vi "Execution End.vi"(8 "error in (no error)":errorcluster, 10 "Execution in":refnum<data-value>, 11 "JsonReportPlugin in":refnum<class "JsonReportPlugin.lvclass">) -> (0 "error out":errorcluster, 2 "Execution out":refnum<data-value>, 3 "JsonReportPlugin out":refnum<class "JsonReportPlugin.lvclass">)   [LabVIEW 2015, in "JsonReportPlugin.lvclass"]
uses:
  JsonReportPlugin.lvclass
  Core/Execution.lvclass
  Core/Step.lvclass
panel:
  out "resulting string":string
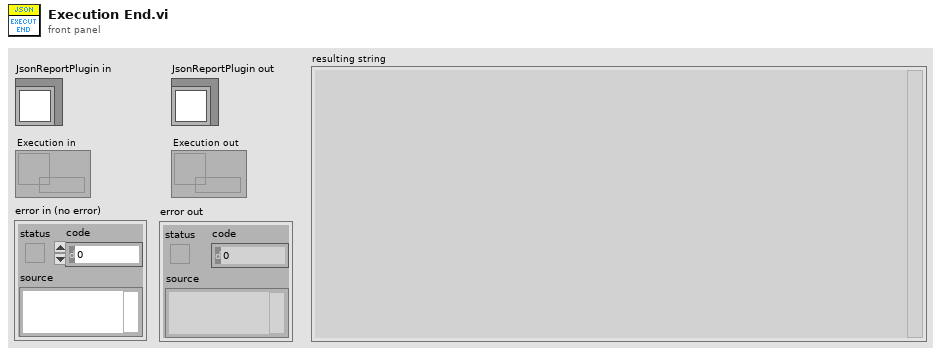
[diagram p1: front panel]
types:
  T1 = typedef "Execution.lvclass/EXECUTION_CONTEXT.ctl" = cluster{"Continue Test":bool, "DUT Info":T2, "StartTime":timestamp, "EndTime":timestamp, "Result":T3, "Info Text":string, "ResultList":T4[]}
  T2 = typedef "Execution.lvclass/DUT_INFO_TYPEDEF.ctl" = cluster{"SN":string, "Model":string, "PartNumber":string, "Revision":string, "Software":string, "Hardware":string}
  T3 = typedef "Execution.lvclass/EXECUTION_RESULT_TYPEDEF.ctl" = enum16{"Unknow", "Terminated", "Passed", "Failed", "Error"}
  T4 = typedef "Execution.lvclass/STEP_RESULT.ctl" = cluster{"StepIndex":u32, "Step":refnum<class "Step.lvclass">, "StartTime":timestamp, "EndTime":timestamp, "Result":T5, "Error Info":string, "Measure Results":T6[]}
  T5 = typedef "Step.lvclass/STEP_STATUS.ctl" = enum16{"Skipped", "Done", "Passed", "Failed", "Error"}
  T6 = typedef "Execution.lvclass/STEP_MEASURE_RESULT.ctl" = cluster{"Name":string, "Data Type":T7, "Check Type":T8, "String Limit":string, "Lower Limit":dbl, "Upper Limit":dbl, "Boolean Limit":bool, "Ignore Case":bool, "Measure Data":variant, "Result":T5, "Error Info":string}
  T7 = typedef "Step.lvclass/OUTPUT_DATA_TYPE.ctl" = enum16{"Boolean", "String", "Numeric", "Other"}
  T8 = typedef "Step.lvclass/OUTPUT_CHECK_TYPE.ctl" = enum16{"INVALID", "DO_NOT_CHECK", "RECORD", "VARIABLE", "EQUAL", "NOT_EQUAL", "STR_CONTAINS", "STR_START_WITH", "STR_END_WITH", "STR_REGEX_MATCH", "NUM_GT", "NUM_LT", "NUM_GE", "NUM_LE", "NUM_RANGE", "NUM_RANGE_BDY"}
  T9 = typedef "STATION_INFO_TYPEDEF.ctl" = cluster{"Process":string, "Station Name":string, "Fixture":string, "Production Line":string, "Factory":string}
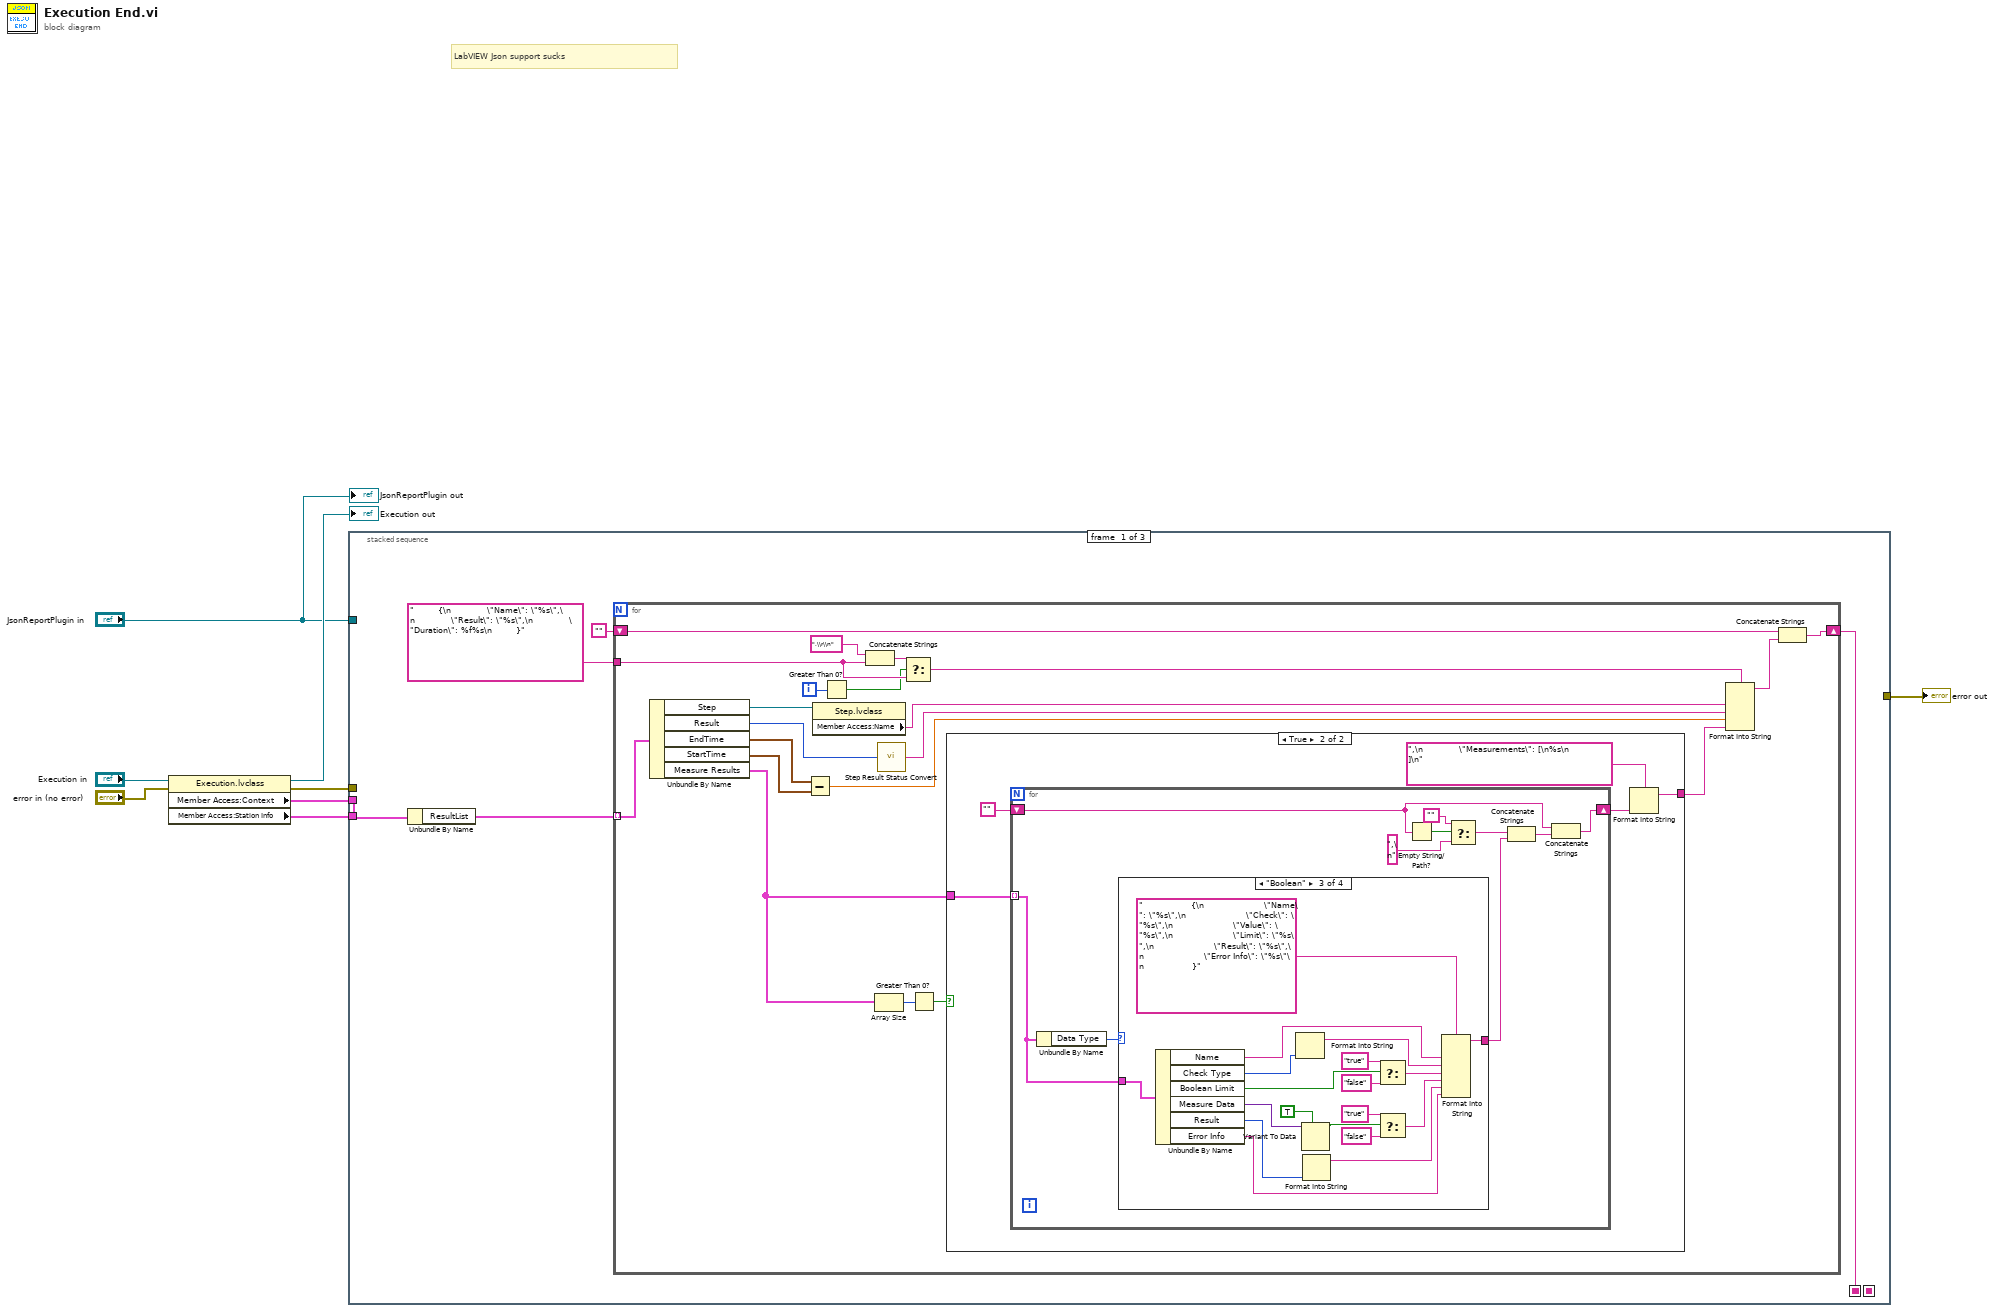
[diagram p0: block diagram]
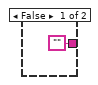
[diagram p2: hidden frame]
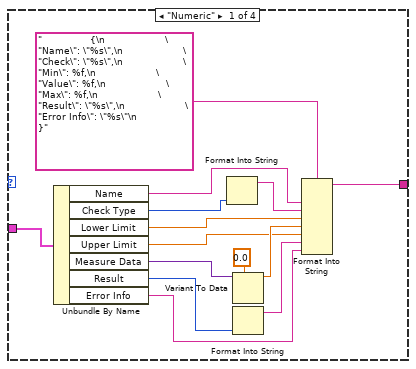
[diagram p3: hidden frame]
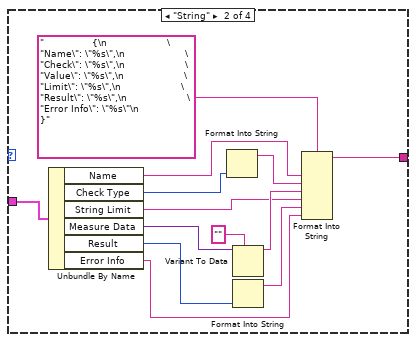
[diagram p4: hidden frame]
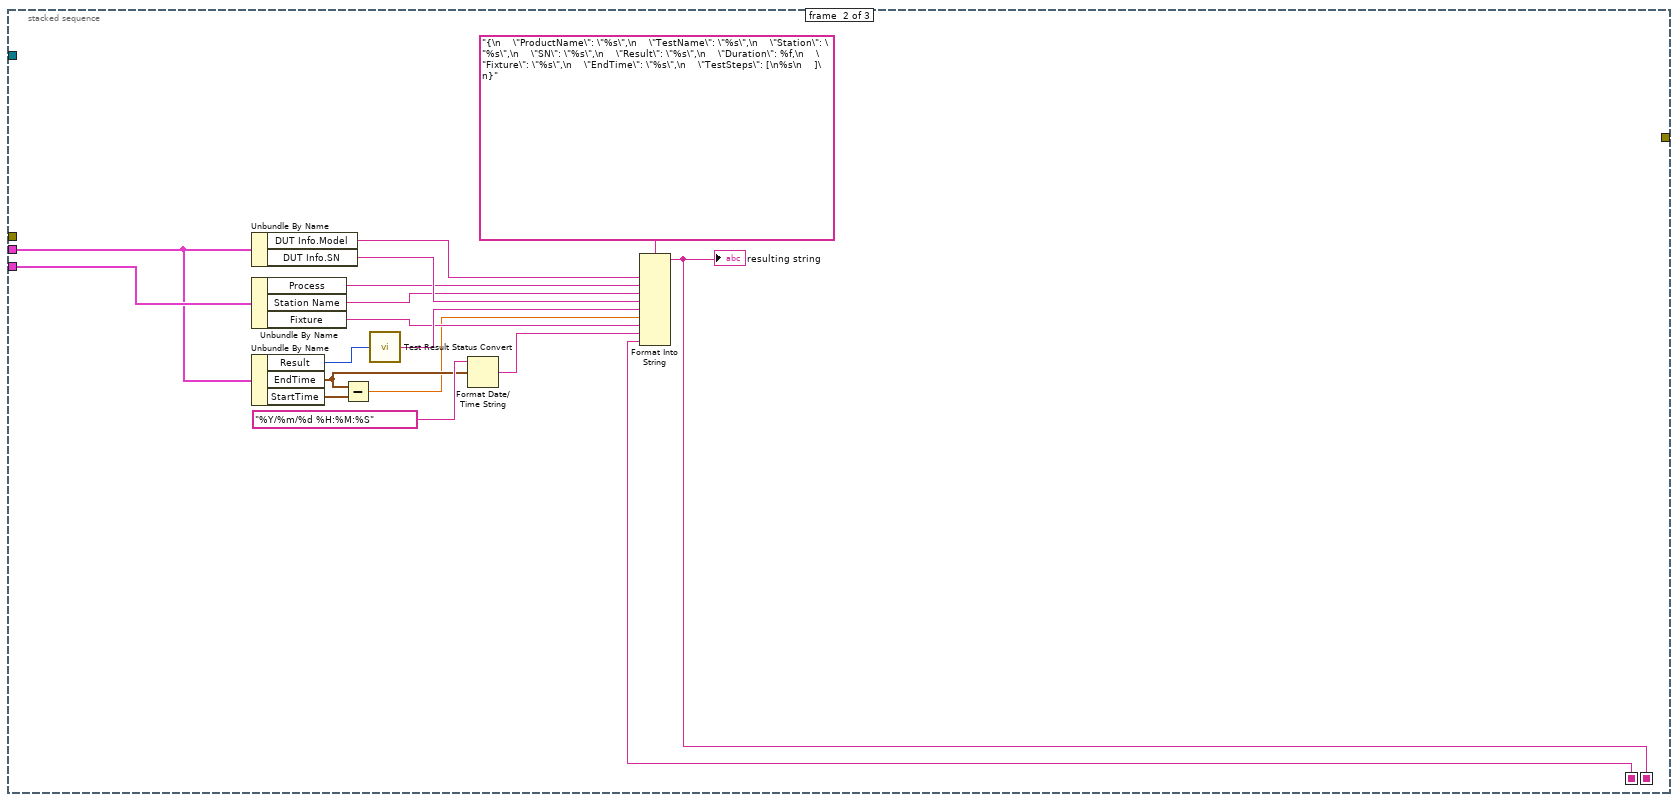
[diagram p6: hidden frame]
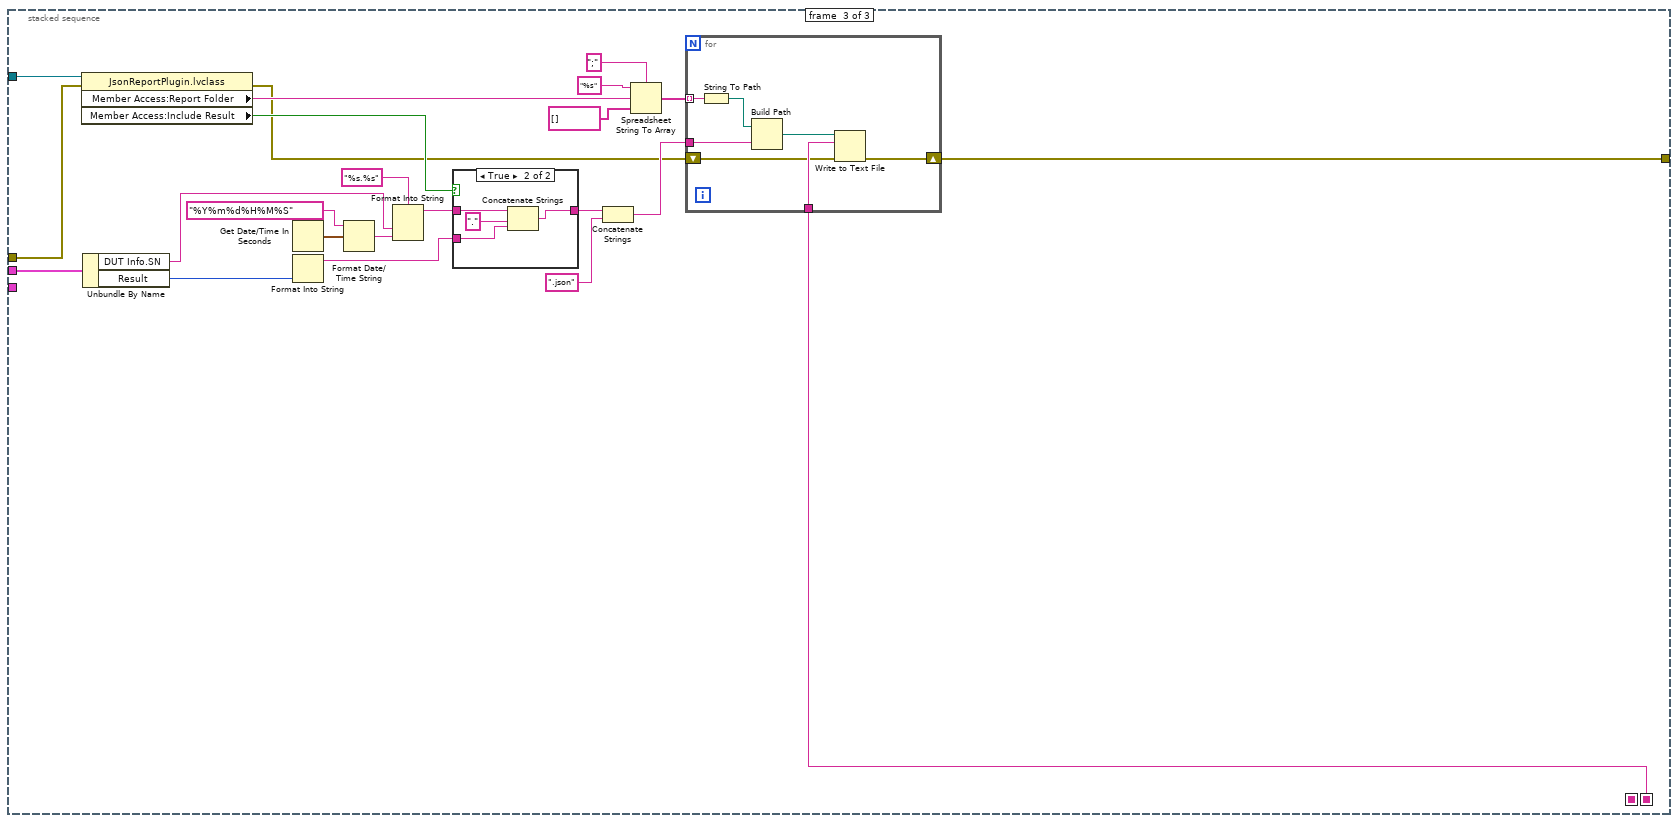
[diagram p7: hidden frame]
diagram:
  # "LabVIEW Json support sucks"
  n1 = property class="Execution.lvclass"(reference="Execution in", error in="error in (no error)") -> (reference out=→"Execution out":refnum<data-value>, error out=w3:errorcluster, "Member Access:Context"=w6:T1, "Member Access:Station Info"=w5:T9)
  n2 = stacked-sequence {
    seq-local: [w9 _ _] -> [_ w99 _]
    seq-local: [_ w97 _] -> [_ _ w116]
    tunnel: w6 -> [w13 w100 w115]
    tunnel: w5 -> [_ w101 _]
    tunnel: "JsonReportPlugin in" -> [_ _ w118]
    tunnel: w3 -> [_ _ w117]
    tunnel: [_ _ w114] -> w1
    frame #0 {
      n3 = Unbundle By Name(w13) -> ("ResultList"=w12:T4[])
      n4 = for {
        tunnel: w12 -> [w34] mode=indexing
        tunnel: "        {\n            \"Name\": \"%s\",\n            \"Result\": \"%s\",\n            \"Duration\": %f%s\n        }" -> [w30]
        shift-right: [w20] -> w9
        shift-left: "" -> [w22]
        i -> [w33]
        n5 = Unbundle By Name(w34) -> ("Step"=w27:refnum<class "Step.lvclass">, "Result"=w18:T5, "EndTime"=w25:timestamp, "StartTime"=w24:timestamp, "Measure Results"=w16:T6[])
        n6 = Subtract(x=w25, y=w24) -> (x-y=w23:dbl)
        n7 = property class="Step.lvclass"(reference=w27) -> ("Member Access:Name"=w26:string)  [unwired: 1 in, 2 out]
        n8 = Greater Than 0?(x=w33) -> (x > 0?=w29:bool)
        n9 = Concatenate Strings(",\\r\\n", w30) -> (w31:string)
        n10 = Array Size(array=w16) -> (size(s)=w15:i32)
        n11 = call "Step Result Status Convert.vi"("Result"=w18) -> ("Result String"=w17:string)
        n12 = Select(t=w31, s=w29, f=w30) -> (s? t:f=w28:string)
        n13 = Greater Than 0?(x=w15) -> (x > 0?=w14:bool)
        n14 = case shown="True" w14 {
          tunnel: ["" w37] -> w19
          tunnel: w16 -> [_ w39]
          frame False {
          }
          frame True {
            n15 = for {
              tunnel: w39 -> [w41] mode=indexing
              shift-right: [w50] -> w38
              shift-left: "" -> [w49]
              n16 = Unbundle By Name(w41) -> ("Data Type"=w43:T7)
              n17 = case shown="\"Boolean\"" w43 {
                tunnel: w41 -> [w63 w76 w95 _]
                tunnel: [w58 w74 w93 _] -> w42
                frame "Numeric" {
                  n18 = Unbundle By Name(w63) -> ("Name"=w55:string, "Check Type"=w57:T8, "Lower Limit"=w61:dbl, "Upper Limit"=w59:dbl, "Measure Data"=w54:variant, "Result"=w53:T5, "Error Info"=w51:string)
                  n19 = Format Into String(w57) -> (resulting string=w56:string)  [unwired: 3 in, 1 out]
                  n20 = Variant To Data(type=0.0 ("Upper Limit"), Variant=w54) -> (data=w60:dbl)  [unwired: 1 in, 1 out]
                  n21 = Format Into String(w53) -> (resulting string=w52:string)  [unwired: 3 in, 1 out]
                  n22 = Format Into String(format string="                {\n                    \"Name\": \"%s\",\n                    \"Check\": \"%s\",\n                    \"Min\": %f,\n                    \"Value\": %f,\n                    \"Max\": %f,\n                    \"Result\": \"%s\",\n                    \"Error Info\": \"%s\"\n                }", w55, w56, w61, w60, w59, w52, w51) -> (resulting string=w58:string)  [unwired: 2 in, 1 out]
                }
                frame "String" {
                  n23 = Unbundle By Name(w76) -> ("Name"=w71:string, "Check Type"=w73:T8, "String Limit"=w69:string, "Measure Data"=w68:variant, "Result"=w67:T5, "Error Info"=w65:string)
                  n24 = Format Into String(w73) -> (resulting string=w72:string)  [unwired: 3 in, 1 out]
                  n25 = Variant To Data(type="" ("Upper Limit"), Variant=w68) -> (data=w70:string)  [unwired: 1 in, 1 out]
                  n26 = Format Into String(w67) -> (resulting string=w66:string)  [unwired: 3 in, 1 out]
                  n27 = Format Into String(format string="                {\n                    \"Name\": \"%s\",\n                    \"Check\": \"%s\",\n                    \"Value\": \"%s\",\n                    \"Limit\": \"%s\",\n                    \"Result\": \"%s\",\n                    \"Error Info\": \"%s\"\n                }", w71, w72, w70, w69, w66, w65) -> (resulting string=w74:string)  [unwired: 2 in, 1 out]
                }
                frame "Boolean" {
                  n28 = Unbundle By Name(w95) -> ("Name"=w90:string, "Check Type"=w92:T8, "Boolean Limit"=w87:bool, "Measure Data"=w81:variant, "Result"=w80:T5, "Error Info"=w78:string)
                  n29 = Format Into String(w92) -> (resulting string=w91:string)  [unwired: 3 in, 1 out]
                  n30 = Variant To Data(type=TRUE, Variant=w81) -> (data=w82:bool)  [unwired: 1 in, 1 out]
                  n31 = Format Into String(w80) -> (resulting string=w79:string)  [unwired: 3 in, 1 out]
                  n32 = Select(t="true", s=w87, f="false") -> (s? t:f=w86:string)
                  n33 = Select(t="true", s=w82, f="false") -> (s? t:f=w83:string)
                  n34 = Format Into String(format string="                {\n                    \"Name\": \"%s\",\n                    \"Check\": \"%s\",\n                    \"Value\": \"%s\",\n                    \"Limit\": \"%s\",\n                    \"Result\": \"%s\",\n                    \"Error Info\": \"%s\"\n                }", w90, w91, w86, w83, w79, w78) -> (resulting string=w93:string)  [unwired: 2 in, 1 out]
                }
                frame "Other" {
                }
              }
              n35 = Empty String/Path?(string/path=w49) -> (empty?=w44:bool)
              n36 = Select(t="", s=w44, f=",\n") -> (s? t:f=w46:string)
              n37 = Concatenate Strings(w46, w42) -> (w45:string)
              n38 = Concatenate Strings(w49, w45) -> (w50:string)
            }
            n39 = Format Into String(format string=",\n            \"Measurements\": [\n%s\n            ]\n", w38) -> (resulting string=w37:string)  [unwired: 2 in, 1 out]
          }
        }
        n40 = Format Into String(format string=w28, w26, w17, w23, w19) -> (resulting string=w21:string)  [unwired: 2 in, 1 out]
        n41 = Concatenate Strings(w22, w21) -> (w20:string)
      }
    }
    frame #1 {
      n42 = Unbundle By Name(w100) -> ("DUT Info.Model"=w102:string, "DUT Info.SN"=w105:string)
      n43 = Unbundle By Name(w101) -> ("Process"=w103:string, "Station Name"=w104:string, "Fixture"=w108:string)
      n44 = Unbundle By Name(w100) -> ("Result"=w112:T3, "EndTime"=w109:timestamp, "StartTime"=w106:timestamp)
      n45 = Subtract(x=w109, y=w106) -> (x-y=w107:dbl)
      n46 = call "Test Result Status Convert.vi"("Result"=w112) -> ("Result String"=w113:string)
      n47 = Format Date/Time String(time format string (%c)="%Y/%m/%d %H:%M:%S", seconds (now)=w109) -> (date/time string=w110:string)  [unwired: 1 in]
      n48 = Format Into String(format string="{\n    \"ProductName\": \"%s\",\n    \"TestName\": \"%s\",\n    \"Station\": \"%s\",\n    \"SN\": \"%s\",\n    \"Result\": \"%s\",\n    \"Duration\": %f,\n    \"Fixture\": \"%s\",\n    \"EndTime\": \"%s\",\n    \"TestSteps\": [\n%s\n    ]\n}", w102, w103, w104, w105, w113, w107, w108, w110, w99) -> (resulting string=w97:string)  [unwired: 2 in, 1 out]
      "resulting string" <- w97
    }
    frame #2 {
      n49 = property class="JsonReportPlugin.lvclass"(reference=w118, error in=w117) -> (error out=w119:errorcluster, "Member Access:Report Folder"=w121:string, "Member Access:Include Result"=w120:bool)  [unwired: 1 out]
      n50 = Unbundle By Name(w115) -> ("DUT Info.SN"=w125:string, "Result"=w131:T3)
      n51 = Get Date/Time In Seconds() -> (seconds since 1Jan1904=w122:timestamp)
      n52 = Format Into String(w131) -> (resulting string=w134:string)  [unwired: 3 in, 1 out]
      n53 = Format Date/Time String(time format string (%c)="%Y%m%d%H%M%S", seconds (now)=w122) -> (date/time string=w126:string)  [unwired: 1 in]
      n54 = Format Into String(format string="%s.%s", w125, w126) -> (resulting string=w135:string)  [unwired: 2 in, 1 out]
      n55 = case shown="True" w120 {
        tunnel: w134 -> [_ w139]
        tunnel: w135 -> [w137 w141]
        tunnel: [w137 w138] -> w136
        frame False {
        }
        frame True {
          n56 = Concatenate Strings(w141, ".", w139) -> (w138:string)
        }
      }
      n57 = Concatenate Strings(w136, ".json") -> (w133:string)
      n58 = Spreadsheet String To Array(delimiter (Tab)=";", format string="%s", spreadsheet string=w121, array type (2D Dbl)=string[] []) -> (array=w130:string[])
      n59 = for {
        tunnel: w133 -> [w148]
        tunnel: w116 -> [w146]
        tunnel: w130 -> [w143] mode=indexing
        shift-right: [w144] -> w114
        shift-left: w119 -> [w145]
        n60 = String To Path(string=w143) -> (path=w142:path)
        n61 = Build Path(base path=w142, name or relative path=w148) -> (appended path=w147:path)
        n62 = Write to Text File(file (use dialog)=w147, text=w146, error in=w145) -> (error out=w144:errorcluster)  [unwired: 1 in, 2 out]
      }
    }
  }
  "error out" <- w1
  "JsonReportPlugin out" <- "JsonReportPlugin in"
